vi "Enter Button Event.vi"(8 "error in (no error)":errorcluster, 10 "Variant":variant, 11 "ATM Data":T1={"UI Refs"={"Right Buttons"=refnum, "Left Buttons"=refnum, "User Input"=refnum, "ATM Messages"=refnum, "Left Menu"=refnum, "Right Menu"=refnum, "Enter"=refnum}, "Map"={}, "Login Valid?"=FALSE, "Queue Message"=refnum, "State"=enum."None", "User"={"Pin"="", "First Name"="", "Last Name"="", "Balance"=0.0, "Login Valid?"=FALSE}, "Main States"={"Message"="Initialize", "Data"=variant}}) -> (0 "error out":errorcluster, 3 "ATM Data Out":T1={"UI Refs"={"Right Buttons"=refnum, "Left Buttons"=refnum, "User Input"=refnum, "ATM Messages"=refnum, "Left Menu"=refnum, "Right Menu"=refnum, "Enter"=refnum}, "Map"={}, "Login Valid?"=FALSE, "Queue Message"=refnum, "State"=enum."None", "User"={"Pin"="", "First Name"="", "Last Name"="", "Balance"=0.0, "Login Valid?"=FALSE}, "Main States"={"Message"="Initialize", "Data"=variant}})   [LabVIEW 2020, in "ATM Machine.lvlib"]
uses:
  ATM Machine.lvlib
  Cluster - ATM Machine Data.ctl
  Users/khemr/OneDrive/Desktop/Labview Training/CLD/New ATM_KR/ATM Machine/Cluster - Message Cluster.ctl
  Enum - ATM States.ctl
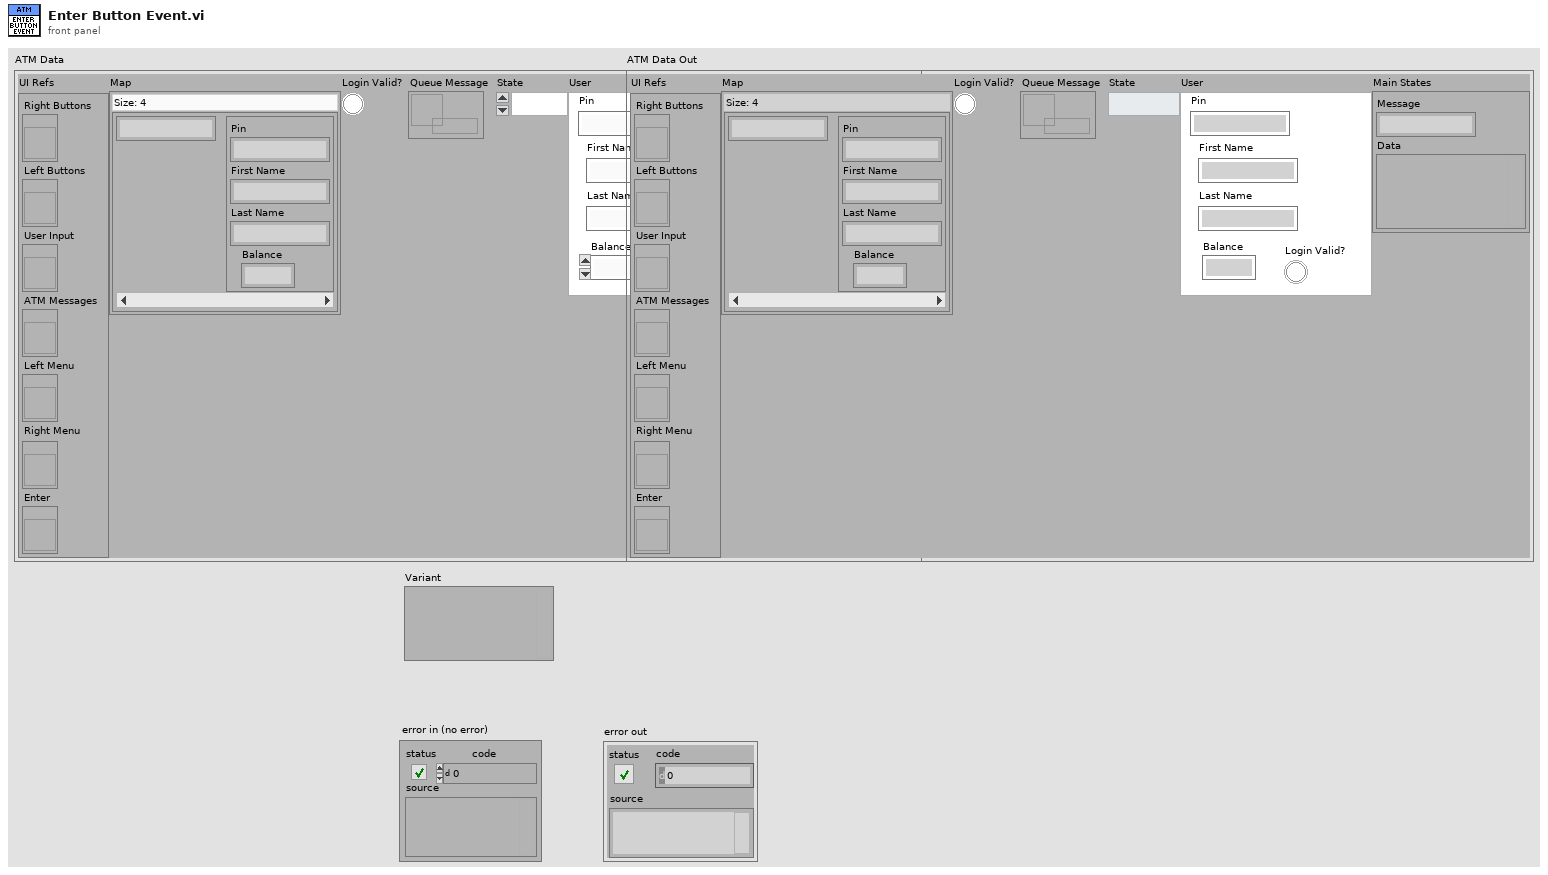
[diagram p1: front panel]
types:
  T1 = typedef "ATM Machine.lvlib/Cluster - ATM Machine Data.ctl" = cluster{"UI Refs":cluster{"Right Buttons":refnum<vi>, "Left Buttons":refnum<vi>, "User Input":refnum<vi>, "ATM Messages":refnum<vi>, "Left Menu":refnum<vi>, "Right Menu":refnum<vi>, "Enter":refnum<vi>}, "Map":map{string, cluster{"Pin":string, "First Name":string, "Last Name":string, "Balance":dbl}}, "Login Valid?":bool, "Queue Message":refnum<queue>, "State":T2, "User":cluster{"Pin":string, "First Name":string, "Last Name":string, "Balance":dbl, "Login Valid?":bool}, "Main States":cluster{"Message":string, "Data":variant}}
  T2 = typedef "ATM Machine.lvlib/Enum - ATM States.ctl" = enum16{"None", "Deposit", "Withdraw", "Card Inserted", "Balance Inquiry", "Return Card and Terminate", "Fast Cash"}
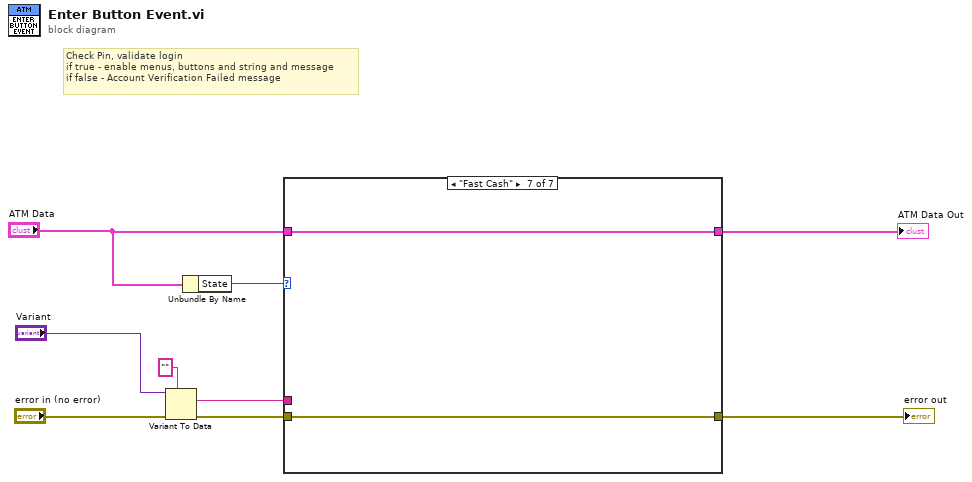
[diagram p0: block diagram]
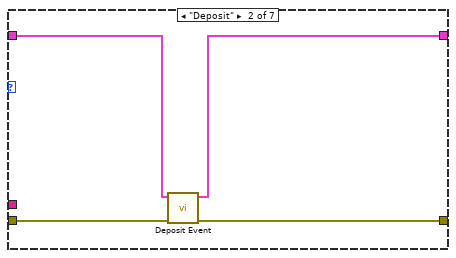
[diagram p3: hidden frame]
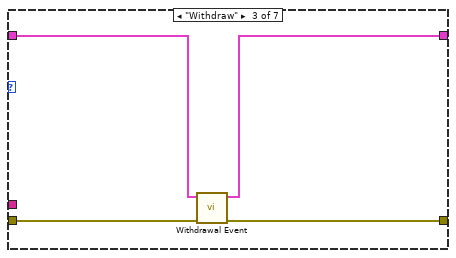
[diagram p4: hidden frame]
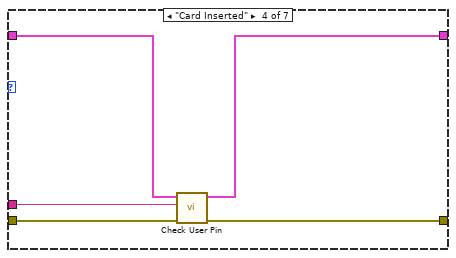
[diagram p5: hidden frame]
diagram:
  # "Check Pin, validate login\nif true - enable menus, buttons and string and message\nif false - Account Verification Failed message"
  n1 = Variant To Data(error in="error in (no error)", type="", Variant="Variant") -> (data=w1:string, error out=w4:errorcluster)
  n2 = Unbundle By Name("ATM Data") -> ("State"=w6:T2)
  n3 = case shown="\"Fast Cash\"" w6 {
    tunnel: [w11 w13 w19 w24 w26 w28 w30] -> w9
    tunnel: w4 -> [w11 w14 w18 w23 w26 w28 w30]
    tunnel: [w10 w15 w17 w22 w25 w27 w29] -> w8
    tunnel: "ATM Data" -> [w10 w12 w16 w21 w25 w27 w29]
    tunnel: w1 -> [_ _ _ w20 _ _ _]
    frame "None", Default {
    }
    frame "Deposit" {
      n4 = call "Deposit Event.vi"("error in"=w14, "ATM Data"=w12) -> ("error out"=w13:errorcluster, "ATM Data Out"=w15:T1)  [unwired: 8 in]
    }
    frame "Withdraw" {
      n5 = call "Withdrawal Event.vi"("error in"=w18, "ATM Data"=w16) -> ("error out"=w19:errorcluster, "ATM Data Out"=w17:T1)  [unwired: 8 in]
    }
    frame "Card Inserted" {
      n6 = call "Check User Pin.vi"("error in (no error)"=w23, "User Pin"=w20, "ATM Data"=w21) -> ("error out"=w24:errorcluster, "ATM Data Out"=w22:T1)  [unwired: 7 in]
    }
    frame "Balance Inquiry" {
    }
    frame "Return Card and Terminate" {
    }
    frame "Fast Cash" {
    }
  }
  "error out" <- w9
  "ATM Data Out" <- w8
